vi "Initialization VI.vi"(8 "error in (no error)":errorcluster, 10 "Custom XML":string, 11 "Device Item Ref in":T1 format="%.0x") -> (0 "error out":errorcluster, 3 "Device Item Ref out":T1 format="%.0x")   [LabVIEW 2014, in "CAN Bus Monitor System Explorer.lvlib"]
uses:
  CAN Bus Monitor System Explorer.lvlib
  <vilib>/NI Veristand/Custom Device API/Custom Device Item Ref.ctl
  <vilib>/NI Veristand/Custom Device API/Custom Device Channel.ctl
  <vilib>/NI Veristand/Custom Device API/Custom Device Channel Type.ctl
  <vilib>/NI Veristand/Custom Device API/Custom Device API.lvlib
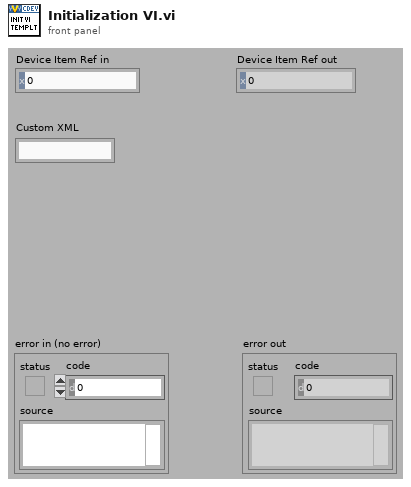
[diagram p1: front panel]
types:
  T1 = typedef "Custom Device API.lvlib/Custom Device Item Ref.ctl" = u64
  T2 = typedef "Custom Device API.lvlib/Custom Device Channel.ctl" = cluster{"Type":T3, "Units":string, "Default Value":dbl, "Faultable":bool, "Scalable":bool}
  T3 = typedef "Custom Device API.lvlib/Custom Device Channel Type.ctl" = enum16{"Input", "Output"}
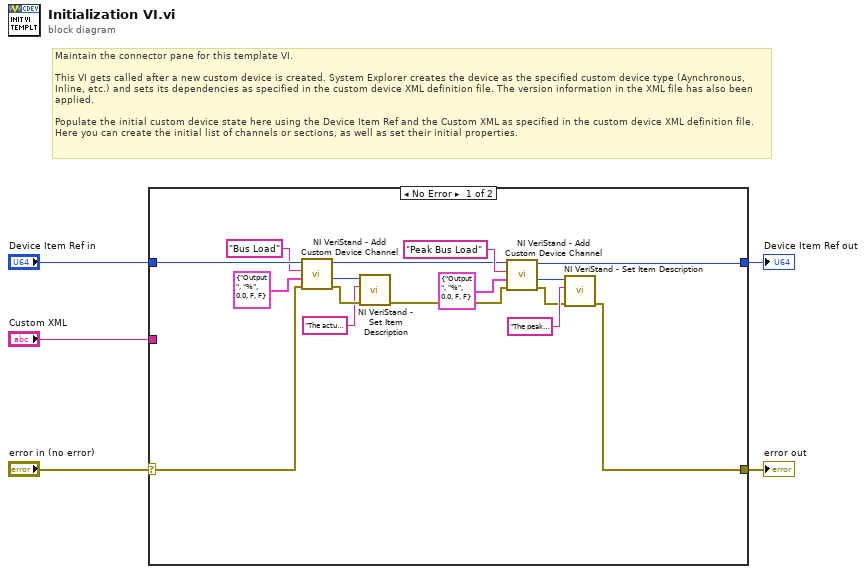
[diagram p0: block diagram]
diagram:
  # "Maintain the connector pane for this template VI.\n\nThis VI gets called after a new custom device is created. System Explorer creates the device as the specified custom device type (Aynchronous, Inline, etc.) and sets its dependencies as specified in the custom device XML definition file. The version information in the XML file has also been applied.\n\nPopulate the initial custom device state here using the Device Item Ref and the Custom XML as specified in the custom device XML definition file. Here you can create the initial list of channels or sections, as well as set their initial properties."
  n1 = case shown="No Error" "error in (no error)" {
    selector: "error in (no error)" -> [w16 w23]
    tunnel: [w7 w23] -> w5
    tunnel: [w6 w22] -> w3
    tunnel: "Device Item Ref in" -> [w21 w22]
    tunnel: "Custom XML" -> [_ _]
    frame No Error {
      n2 = call <vilib>:"NI VeriStand - Add Custom Device Channel.vi"("error in (no error)"=w16, "Channel"=T2 {"Type"=enum."Output", "Units"="%", "Default Value"=0.0, "Faultable"=FALSE, "Scalable"=FALSE}, "Channel Name"="Bus Load", "Parent Ref in"=w21) -> ("error out"=w17:errorcluster, "Channel Ref"=w18:T1, "Parent Ref out"=w9:T1)  [unwired: 4 in, 1 out]
      n3 = call <vilib>:"NI VeriStand - Set Item Description.vi"("error in (no error)"=w17, "Description"="The actual calculated CAN Bus Load in percent.", "Item Ref in"=w18) -> ("error out"=w8:errorcluster)  [unwired: 6 in, 2 out]
      n4 = call <vilib>:"NI VeriStand - Add Custom Device Channel.vi"("error in (no error)"=w8, "Channel"=T2 {"Type"=enum."Output", "Units"="%", "Default Value"=0.0, "Faultable"=FALSE, "Scalable"=FALSE}, "Channel Name"="Peak Bus Load", "Parent Ref in"=w9) -> ("error out"=w13:errorcluster, "Channel Ref"=w12:T1, "Parent Ref out"=w6:T1)  [unwired: 4 in, 1 out]
      n5 = call <vilib>:"NI VeriStand - Set Item Description.vi"("error in (no error)"=w13, "Description"="The peak CAN bus load since the start of measurement.", "Item Ref in"=w12) -> ("error out"=w7:errorcluster)  [unwired: 6 in, 2 out]
    }
    frame Error {
    }
  }
  "error out" <- w5
  "Device Item Ref out" <- w3
